vi "CTRE_Phoenix_CANdle_SetStatusFrameRate.vi"(6 "timeoutMs":u32, 8 "error in (no error)":errorcluster, 9 "Period (ms)":u8, 10 "CANdle Status Frame":T1=267264 items=["Status_1_General"=267264, "Status_2_Startup"=267328, "Status_3_FirmwareApiStatus"=267392, "Status_4_ControlTelem"=267456, "Status_5_PixelPulseTrain"=267520, "Status_6_BottomPixels"=267584, "Status_7_TopPixels"=267648], 11 "CTRE_CANdle_DeviceRef":T2) -> (0 "error out":errorcluster, 3 "CTRE_CANdle_DeviceRef":T2)   [LabVIEW 2020]
doc: "<b>Period (ms)</b> sets the rate at which Status Data is sent."
uses:
  <vilib>/Rock Robotics/WPI/ThirdParty/Phoenix-LabVIEW/CANdle/Controls/CTRE_Phoenix_CANdle_DeviceRef.ctl
  <vilib>/Rock Robotics/WPI/ThirdParty/Phoenix-LabVIEW/CANdle/Controls/CTRE_Phoenix_CANdle_StatusFrame.ctl
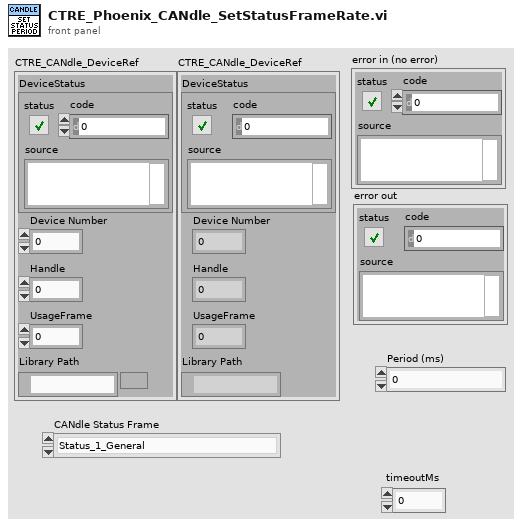
[diagram p1: front panel]
types:
  T1 = typedef "CTRE_Phoenix_CANdle_StatusFrame.ctl" = u32
  T2 = typedef "CTRE_Phoenix_CANdle_DeviceRef.ctl" = cluster{"DeviceStatus":errorcluster, "Device Number":u8, "Handle":u64, "UsageFrame":u32, "Library Path":path}
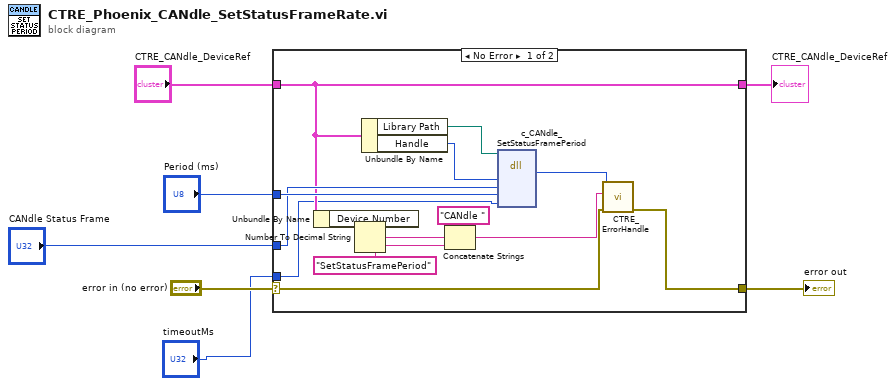
[diagram p0: block diagram]
diagram:
  n1 = case shown="No Error" "error in (no error)" {
    selector: "error in (no error)" -> [w10 w22]
    tunnel: [w9 w22] -> w6
    tunnel: [w12 w23] -> w2
    tunnel: "CTRE_CANdle_DeviceRef" -> [w12 w23]
    tunnel: "Period (ms)" -> [w19 _]
    tunnel: "CANdle Status Frame" -> [w18 _]
    tunnel: "timeoutMs" -> [w8 _]
    frame No Error {
      n2 = Unbundle By Name(w12) -> ("Device Number"=w16:u8)
      n3 = Number To Decimal String(number=w16) -> (decimal integer string=w15:string)  [unwired: 1 in]
      n4 = Unbundle By Name(w12) -> ("Library Path"=w21:path, "Handle"=w20:u64)
      n5 = Concatenate Strings("CANdle " ("string"), w15, "SetStatusFramePeriod" ("string")) -> (w11:string)
      n6 = dll-call lib="?" fn="c_CANdle_SetStatusFramePeriod"(path in=w21, "handle"=w20, "statusFrame"=w18, "periodMs"=w19, "timeoutms"=w8) -> ("return type"=w17:i32)  [unwired: 6 in, 2 out]
      n7 = call <vilib>:"CTRE_ErrorHandle.vi"("error in"=w10, "origin"=w11, "code"=w17) -> ("error out"=w9:errorcluster)  [unwired: 8 in]
    }
    frame Error {
    }
  }
  "error out" <- w6
  "CTRE_CANdle_DeviceRef" <- w2
